vi "calculate_hexahedron_area.vi"(11 "Dimentions":T1) -> (3 "Area of hexahedron":dbl)   [LabVIEW 2022 SP3]
uses:
  Dimensions_input_tdef.ctl
panel:
  in  "error in":errorcluster
  out "error out":errorcluster
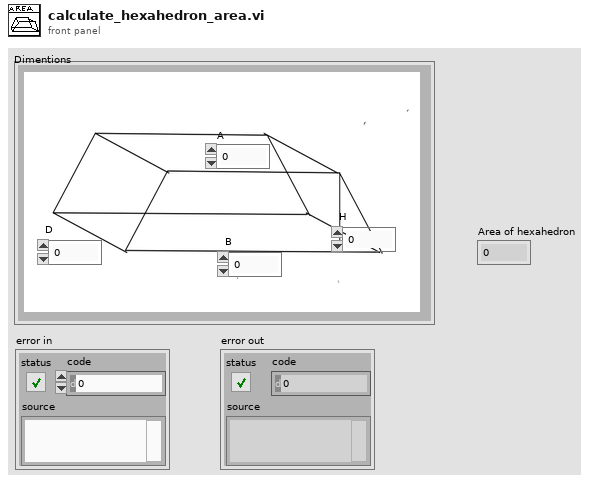
[diagram p1: front panel]
types:
  T1 = typedef "Dimensions_input_tdef.ctl" = cluster{"B":dbl, "A":dbl, "H":dbl, "D":dbl}
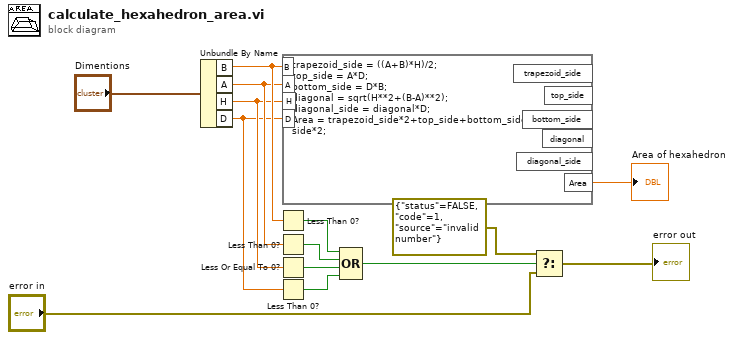
[diagram p0: block diagram]
diagram:
  n1 = Unbundle By Name("Dimentions") -> ("B"=w12:dbl, "A"=w11:dbl, "H"=w10:dbl, "D"=w9:dbl)
  n2 = Less Than 0?(x=w12) -> (x < 0?=w8:bool)
  n3 = Less Than 0?(x=w11) -> (x < 0?=w7:bool)
  n4 = Less Or Equal To 0?(x=w10) -> (x <= 0?=w6:bool)
  n5 = Less Than 0?(x=w9) -> (x < 0?=w5:bool)
  n6 = formula code="trapezoid_side = ((A+B)*H)/2;\ntop_side = A*D;\nbottom_side = D*B;\ndiagonal = sqrt(H**2+(B-A)**2);\ndiagonal_side = diagonal*D;\nArea = trapezoid_side*2+top_side+bottom_side+diagonal_side*2;"("B"=w12, "A"=w11, "H"=w10, "D"=w9) -> ("Area"=→"Area of hexahedron":dbl)  [unwired: 5 out]
  n7 = Compound Arithmetic op=OR(w8, w7, w6, w5) -> (w4:bool)
  n8 = Select(t=errorcluster {"status"=FALSE, "code"=1, "source"="invalid number"} ("error constant"), s=w4, f="error in") -> (s? t:f=→"error out":errorcluster)
